vi "targetSelector.vi"(5 "Longitude":dbl, 7 "Latitude":dbl, 9 "New Target":T1(plugin-control), 11 "Existing Targets":T2(array[cluster]) {"Orientation" items=["North", "North-East", "East", "South-East", "South", "South-West", "West", "North-West"]}) -> (0 "cancelled":bool, 1 "imageSelect 2":bool, 3 "index":u32)   [LabVIEW 2014]
panel:
  in  "imageSelect":bool
  in  "select":bool
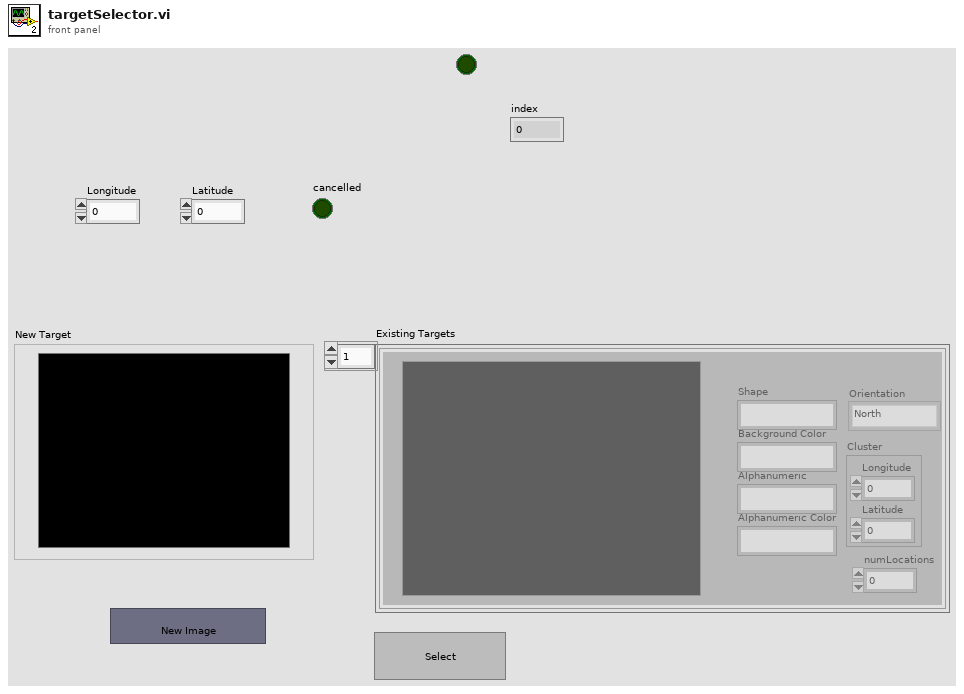
[diagram p1: front panel]
types:
  T1 = typedef "IMAQ Image.ctl" = refnum<image>
  T2 = cluster{"Image Out":T1, "Shape":string, "Background Color":string, "Alphanumeric":string, "Alphanumeric Color":string, "Cluster":cluster{"Longitude":dbl, "Latitude":dbl}, "Orientation":u16, "numLocations":i32}[]
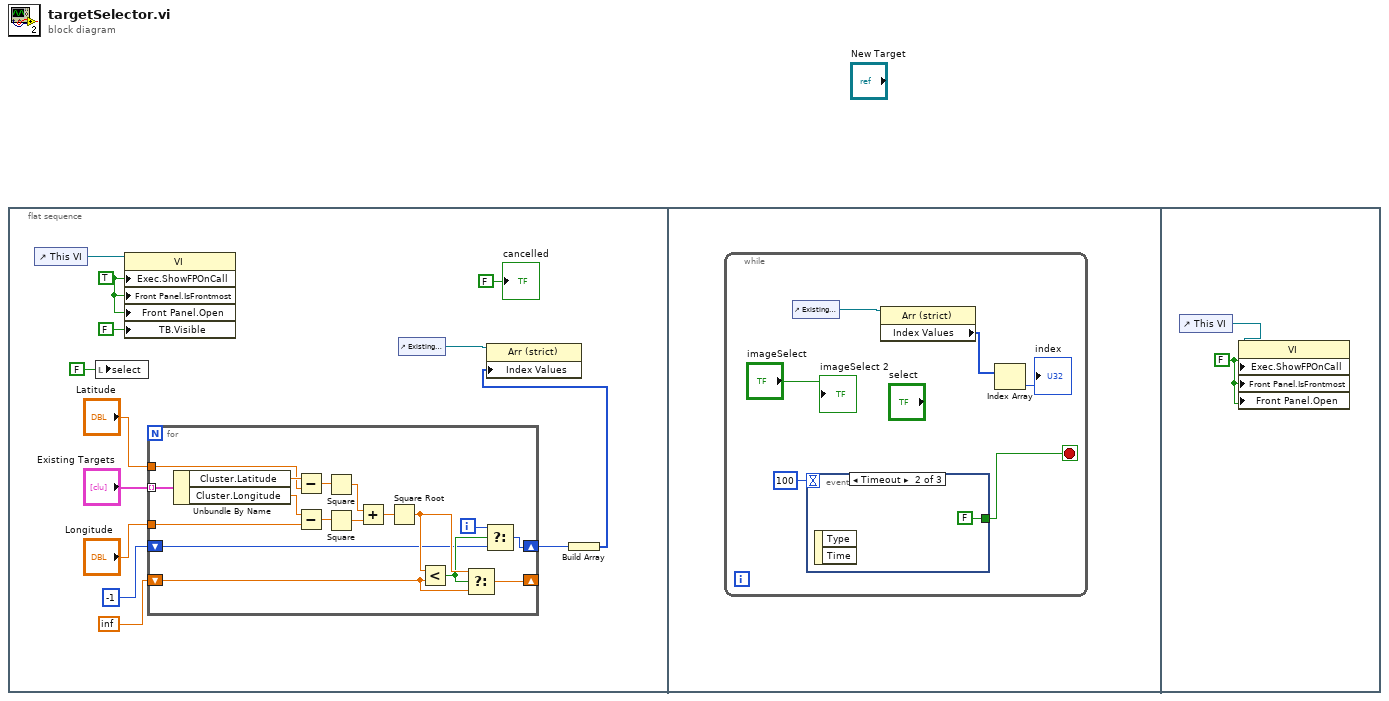
[diagram p0: block diagram]
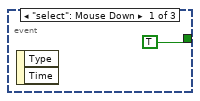
[diagram p2: hidden frame]
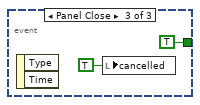
[diagram p3: hidden frame]
diagram:
  n1 = flat-sequence {
    frame #0 {
      w12 = TRUE ("Execution:Show Front Panel On Call")
      n2 = control-ref of="This VI"() -> (w11:refnum<vi>)
      n3 = local write "select"(FALSE ("select")) -> ()
      n4 = property class="VI"(reference=w11, "Exec.ShowFPOnCall"=w12, "Front Panel.IsFrontmost"=w12, "Front Panel.Open"=w12, "TB.Visible"=FALSE ("Tool Bar:Visible")) -> ()  [unwired: 1 in, 2 out]
      n5 = for {
        tunnel: "Existing Targets" -> [w30] mode=indexing
        tunnel: "Latitude" -> [w28]
        tunnel: "Longitude" -> [w26]
        shift-right: [w20] -> _
        shift-left: inf -> [w18]
        shift-right: [w15] -> w3
        shift-left: -1 -> [w14]
        i -> [w16]
        n6 = Unbundle By Name(w30) -> ("Cluster.Latitude"=w29:dbl, "Cluster.Longitude"=w27:dbl)
        n7 = Subtract(x=w29, y=w28) -> (x-y=w24:dbl)
        n8 = Subtract(x=w27, y=w26) -> (x-y=w25:dbl)
        n9 = Square(x=w24) -> (x^2=w23:dbl)
        n10 = Square(x=w25) -> (x^2=w22:dbl)
        n11 = Add(x=w23, y=w22) -> (x+y=w21:dbl)
        n12 = Square Root(x=w21) -> (sqrt(x)=w19:dbl)
        n13 = Less?(x=w19, y=w18) -> (x < y?=w17:bool)
        n14 = Select(t=w19, s=w17, f=w18) -> (s? t:f=w20:dbl)
        n15 = Select(t=w16, s=w17, f=w14) -> (s? t:f=w15:i32)
      }
      n16 = control-ref of="Existing Targets"() -> (w4:refnum<vi>)
      n17 = Build Array(w3) -> (w2:i32[])
      n18 = property class="Arr (strict)"(reference=w4, "Index Values"=w2) -> ()  [unwired: 1 in, 2 out]
      "cancelled" <- FALSE ("cancelled")
    }
    frame #1 {
      n19 = while {
        stop <- w32 stop-if-true
        n20 = control-ref of="Existing Targets"() -> (w36:refnum<vi>)
        n21 = event shown="[1] Timeout" {
          selector: _ -> [_ _ _]
          dyn-events: _ -> [_ _ _]
          timeout: 100 -> [_ _ _]
          tunnel: [TRUE FALSE TRUE] -> w32
          event "select": Mouse Down {
            n22 = event-data() -> ()  [unwired: 1 in, 2 out]
          }
          event Timeout {
            n23 = event-data() -> ()  [unwired: 1 in, 2 out]
          }
          event Panel Close {
            n24 = event-data() -> ()  [unwired: 1 in, 2 out]
            n25 = local write "cancelled"(TRUE ("cancelled")) -> ()
          }
        }
        n26 = property class="Arr (strict)"(reference=w36) -> ("Index Values"=w35:u32[])  [unwired: 1 in, 2 out]
        n27 = Index Array(array=w35) -> (element=→"index":u32)  [unwired: 1 in]
        "imageSelect 2" <- "imageSelect"
      }
    }
    frame #2 {
      w41 = FALSE ("Execution:Show Front Panel On Call")
      n28 = control-ref of="This VI"() -> (w42:refnum<vi>)
      n29 = property class="VI"(reference=w42, "Exec.ShowFPOnCall"=w41, "Front Panel.IsFrontmost"=w41, "Front Panel.Open"=w41) -> ()  [unwired: 1 in, 2 out]
    }
  }
